vi "TEST_of Test Info Dialog.vi"() -> ()   [LabVIEW 2010]
panel:
  out "error out":errorcluster
  out "Cancelled?":bool
  out "Parameter Table Out":string[][](table) caption="Parameter Table + Comment Out"
  in  "ParameterNamesIn":string[](array[string])=["Technician Name", "Part Number", "Serial Number", "Specific Gravity"]
  # "Run This to test the \"Test Information Dialog\"\n1. Enter the names of the fields you want the operator to enter at test time into the ParameterNamesIn array.\n2. When the dialog pops up, you should be able to enter the first field immediately.\n3. <TAB> works to let you enter a value, then TAB, which will take you to the next field (not name). TAB wraps."
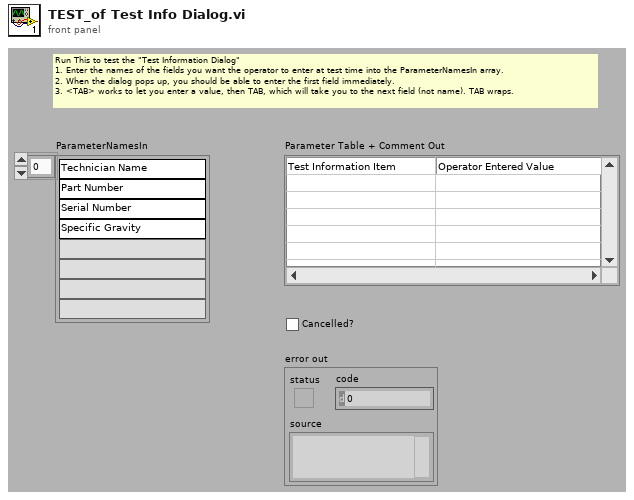
[diagram p1: front panel]
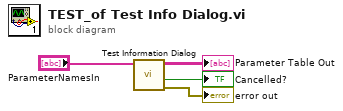
[diagram p0: block diagram]
diagram:
  n1 = call "Test Information Dialog.vi"("ParameterNamesIn"="ParameterNamesIn") -> ("error out"=→"error out":errorcluster, "Cancelled?"=→"Cancelled?":bool, "Parameter Table Out"=→"Parameter Table Out":string[][])  [unwired: 8 in]
